vi "Example Threshold - MoistureReached Callback.vi"(4 "MoistureReached":refnum<user-event>, 5 "Event Data":cluster{"sender":refnum<k24>, "moisture":i32}, 6 "Control Ref":refnum<k24>, 7 "Event Common Data":T1) -> ()   [LabVIEW 2010]
uses:
  C:/tf/play/labview/Tinkerforge.dll
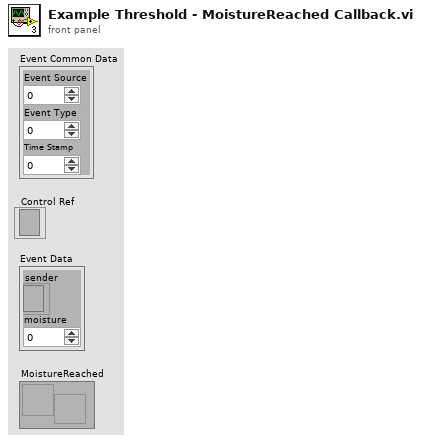
[diagram p1: front panel]
types:
  T1 = cluster{"Event Source":i32, "Event Type":u32, "Time Stamp":u32}
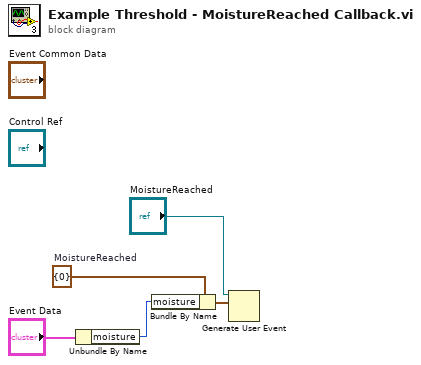
[diagram p0: block diagram]
diagram:
  w5 = cluster{"moisture":i32} {"moisture"=0}  # MoistureReached
  n1 = Unbundle By Name("Event Data") -> ("moisture"=w4:i32)
  n2 = Bundle By Name(cluster=w5, "moisture"=w4) -> (w2:cluster{"moisture":i32})
  n3 = Generate User Event(user event="MoistureReached", event data cluster=w2) -> ()  [unwired: 1 in, 2 out]
